vi "TurnOn.vi"(7 "Voltage Set (V)":dbl, 8 "error in (no error)":errorcluster, 9 "OCP Level (A)":dbl, 10 "OVP Level (V)":dbl, 11 "PSU in":refnum<class "PSU.lvclass">) -> (0 "error out":errorcluster, 3 "PSU out":refnum<class "PSU.lvclass">)   [LabVIEW 2014, in "PSU.lvclass"]
uses:
  PSU.lvclass
  PSU.lvclass/PSU.ctl
  Write On.vi
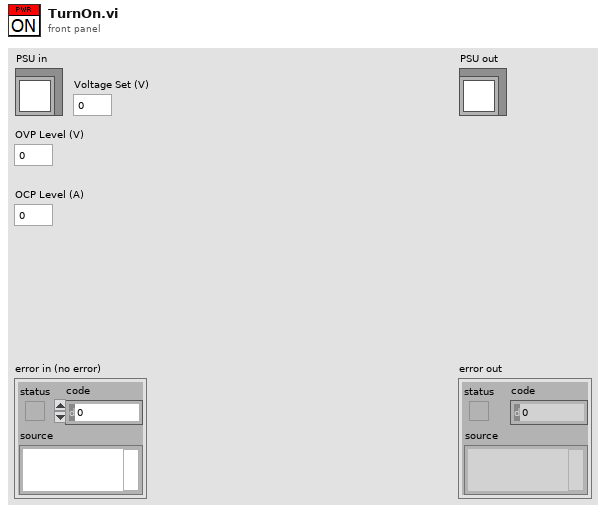
[diagram p1: front panel]
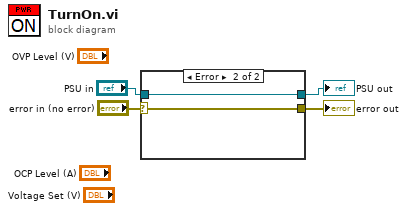
[diagram p0: block diagram]
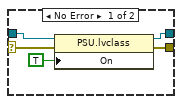
[diagram p2: hidden frame]
diagram:
  n1 = case shown="Error" "error in (no error)" {
    selector: "error in (no error)" -> [w6 w10]
    tunnel: "PSU in" -> [w9 w11]
    tunnel: [w8 w11] -> w2
    tunnel: [w7 w10] -> w1
    frame No Error {
      n2 = property class="PSU.lvclass"(reference=w9, error in=w6, "On"=TRUE) -> (reference out=w8:refnum<class "PSU.lvclass">, error out=w7:errorcluster)
    }
    frame Error {
    }
  }
  "error out" <- w1
  "PSU out" <- w2
